vi "Execution_MessageHanlder_IncrementMessageCounter.vi"(8 "error in (no error)":errorcluster, 11 "MessageHandler in":refnum<class "MessageHandler.lvclass">) -> (0 "error out":errorcluster, 3 "MessageHandler out":refnum<class "MessageHandler.lvclass">)   [LabVIEW 2013, in "MessageHandler.lvclass"]
uses:
  MessageHandler.lvclass
  MessageHandler.lvclass/MessageHandler.ctl
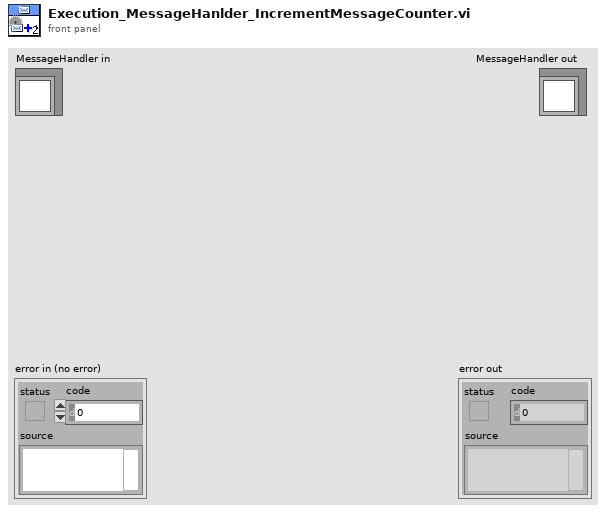
[diagram p1: front panel]
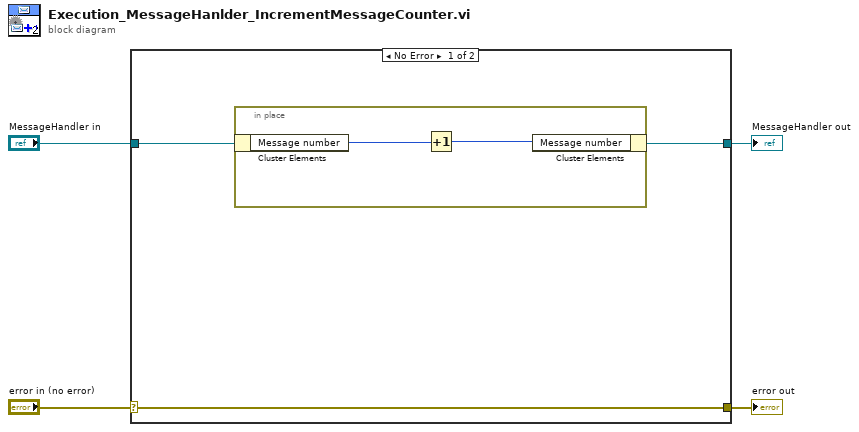
[diagram p0: block diagram]
diagram:
  n1 = case shown="No Error" "error in (no error)" {
    selector: "error in (no error)" -> [w7 w11]
    tunnel: [w7 w11] -> w3
    tunnel: [w5 w10] -> w1
    tunnel: "MessageHandler in" -> [w6 w10]
    frame No Error {
      n2 = in-place {
        n3 = in-place-cluster #1(w6) -> ("Message number"=w9:u32)
        n4 = Increment(x=w9) -> (x+1=w8:u32)
        n5 = in-place-cluster #1("Message number"=w8) -> (w5:refnum<class "MessageHandler.lvclass">)
      }
    }
    frame Error {
    }
  }
  "error out" <- w3
  "MessageHandler out" <- w1
